vi "setDeadband.vi"(8 "Deadband":dbl, 11 "Joystick Axis Value":dbl) -> (3 "Output Motor Value":dbl)   [LabVIEW 2014]
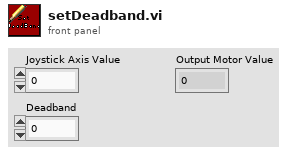
[diagram p1: front panel]
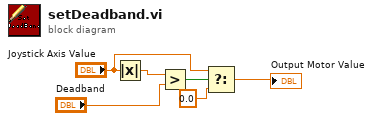
[diagram p0: block diagram]
diagram:
  n1 = Absolute Value(x="Joystick Axis Value") -> (abs(x)=w6:dbl)
  n2 = Greater?(x=w6, y="Deadband") -> (0:w4:bool)
  n3 = Select(t="Joystick Axis Value", s=w4, f=0.0) -> (s? t:f=→"Output Motor Value":dbl)
